vi "Waveform to XY.vi"   [LabVIEW 2019, in "xy_utilities.lvlib"]
doc: "Convert <b>Waveform</b> to <b>XY-data</b>.\n\nWire data to the data input to determine the polymorphic instance to use or manually select the instance."
uses:
  xy_utilities.lvlib
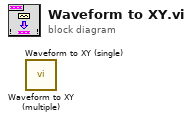
[diagram p0: block diagram]
diagram:
  n1 = call "Waveform to XY (multiple).vi"() -> ()  [unwired: 10 in, 2 out]
  n2 = call "Waveform to XY (single).vi"() -> ()  [unwired: 10 in, 2 out]
